vi "SetV.vi"(8 "error in (no error)":errorcluster, 9 "Chan":i32, 10 "V":dbl, 11 "reference in":refnum<class "PSU_Keysight_34951A.lvclass">) -> (0 "error out":errorcluster, 3 "reference in":refnum<class "PSU_Keysight_34951A.lvclass">)   [LabVIEW 2022 SP3, in "PSU_Keysight_34951A.lvlib" / "PSU_Keysight_34951A.lvclass"]
uses:
  PSU_Keysight_34951A.lvclass
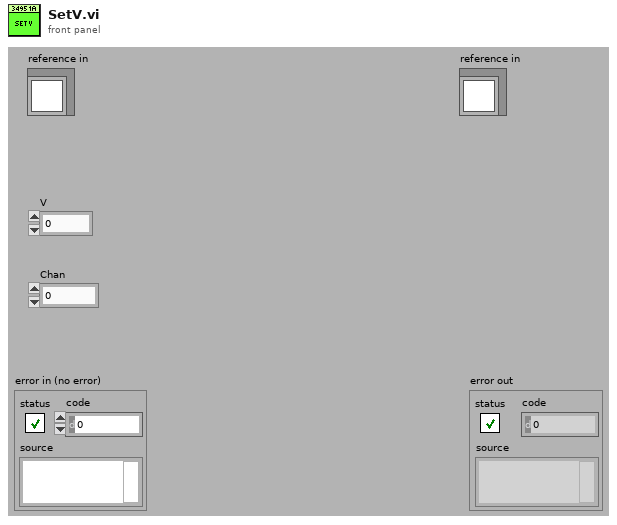
[diagram p1: front panel]
types:
  T1 = typedef "PSU_Keysight_34951A.lvlib/PSU_Keysight_34951A.lvclass/ObjectAttributes.ctl" = cluster{"Config":T2, "VISA res":refnum<visa-resource-name>, "Enabled":bool[], "V":dbl[], "I":dbl[], "Source Type":enum16{"Voltage", "Current"}[]}
  T2 = typedef "PSU_Keysight_34951A.lvlib/PSU_Keysight_34951A.lvclass/Config.ctl" = cluster{"VISA":refnum<visa-resource-name>, "Slot":i32}
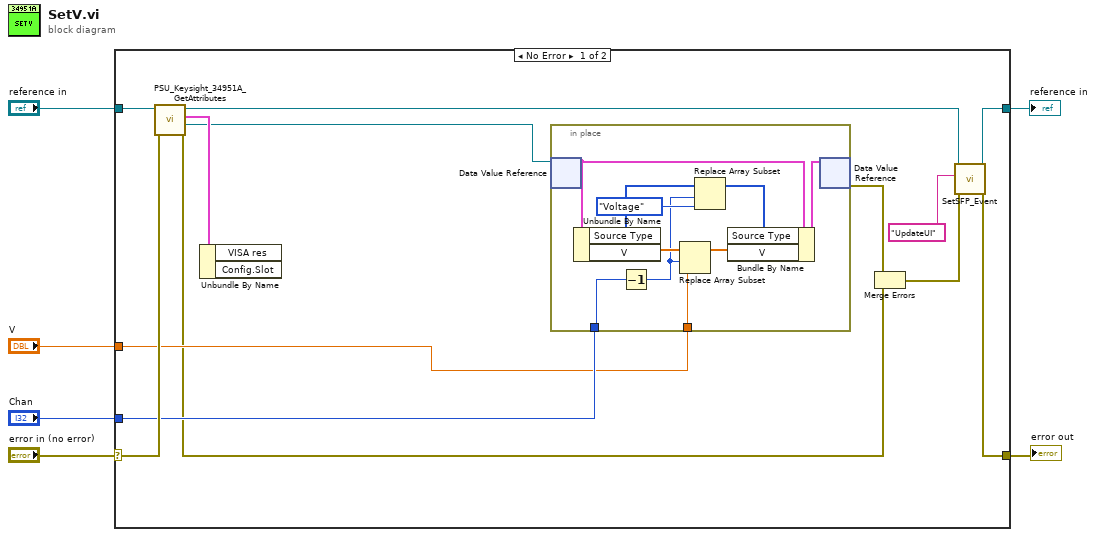
[diagram p0: block diagram]
diagram:
  n1 = case shown="No Error" "error in (no error)" {
    selector: "error in (no error)" -> [w19 w31]
    tunnel: [w9 w31] -> w5
    tunnel: [w10 w30] -> w3
    tunnel: "reference in" -> [w17 w30]
    tunnel: "V" -> [w14 _]
    tunnel: "Chan" -> [w15 _]
    frame No Error {
      n2 = call "PSU_Keysight_34951A_GetAttributes.vi"("error in (no error)"=w19, "reference in"=w17) -> ("error out"=w7:errorcluster, "DataRef"=w16:refnum<data-value>, "Data"=w18:T1, "reference out"=w11:refnum<class "PSU_Keysight_34951A.lvclass">)  [unwired: 6 in]
      n3 = Unbundle By Name(w18) -> ()  [unwired: 2 out]
      n4 = in-place {
        in-place-border: w15 -> [w27]
        in-place-border: w14 -> [w24]
        n5 = in-place-dvr #1(w16) -> (w28:T1)  [unwired: 1 out]
        n6 = Unbundle By Name(w28) -> ("Source Type"=w22:enum16{"Voltage", "Current"}[], "V"=w26:dbl[])
        n7 = Decrement(x=w27) -> (x-1=w20:i32)
        n8 = Replace Array Subset(array=w26, new element=w24, index=w20) -> (w25:dbl[])
        n9 = Replace Array Subset(array=w22, new element=enum16{"Voltage", "Current"}."Voltage" ("new element/subarray"), index=w20) -> (w21:enum16{"Voltage", "Current"}[])
        n10 = Bundle By Name(cluster=w28, "Source Type"=w21, "V"=w25) -> (w29:T1)
        n11 = in-place-dvr #1(w29) -> (w13:errorcluster)  [unwired: 1 out]
      }
      n12 = Merge Errors(w13, w7) -> (w12:errorcluster)
      n13 = call-dynamic "SetSFP_Event.vi"("error in (no error)"=w12, "msg"="UpdateUI" ("Ancestor"), "reference in"=w11) -> ("error out"=w9:errorcluster, "reference out"=w10:refnum<class "PSU_Keysight_34951A.lvclass">)  [unwired: 7 in]
    }
    frame Error {
    }
  }
  "error out" <- w5
  "reference in" <- w3
